vi "Unflatten Asynchronous Execution Units.vi"(8 "error in":errorcluster, 11 "Asynchronous Execution Unit Compiled Information":T4(array[cluster])) -> (0 "error out":errorcluster, 3 "Asynchronous Execution Units":T2(array[cluster]))   [LabVIEW 2020, in "Ballard ARINC 429 Engine.lvlib" / "Custom Device.lvlib"]
uses:
  Custom Device.lvlib
  Asynchronous Execution Unit Compiled Information.ctl
  Asynchronous Execution Unit Runtime Information.ctl
  Interfaces/Execution Unit/Execution Unit.lvclass
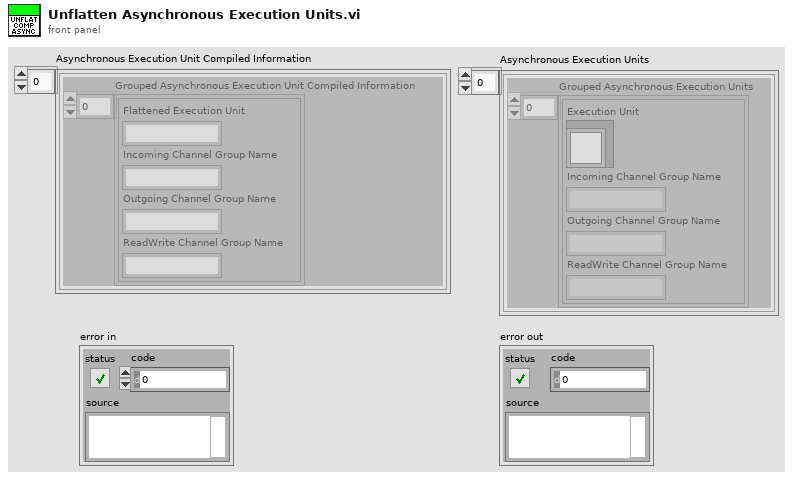
[diagram p1: front panel]
types:
  T1 = typedef "Ballard ARINC 429 Engine.lvlib/Custom Device.lvlib/Asynchronous Execution Unit Runtime Information.ctl" = cluster{"Execution Unit":refnum<class "Execution Unit.lvclass">, "Incoming Channel Group Name":string, "Outgoing Channel Group Name":string, "ReadWrite Channel Group Name":string}
  T2 = cluster{"Grouped Asynchronous Execution Units":T1[]}[]
  T3 = typedef "Ballard ARINC 429 Engine.lvlib/Custom Device.lvlib/Asynchronous Execution Unit Compiled Information.ctl" = cluster{"Flattened Execution Unit":string, "Incoming Channel Group Name":string, "Outgoing Channel Group Name":string, "ReadWrite Channel Group Name":string}
  T4 = cluster{"Grouped Asynchronous Execution Unit Compiled Information":T3[]}[]
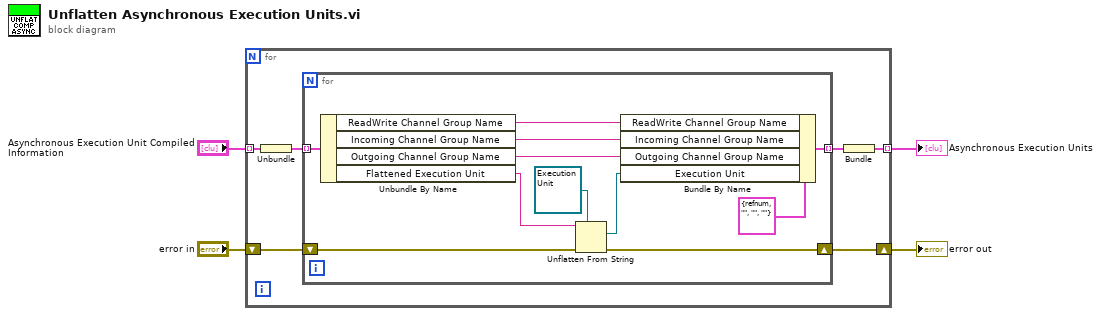
[diagram p0: block diagram]
diagram:
  n1 = for {
    tunnel: "Asynchronous Execution Unit Compiled Information" -> [w8] mode=indexing
    tunnel: [w6] -> w1 mode=indexing
    shift-right: [w9] -> w3
    shift-left: "error in" -> [w10]
    n2 = Unbundle(w8) -> ("Grouped Asynchronous Execution Unit Compiled Information"=w7:T3[])
    n3 = for {
      tunnel: w7 -> [w18] mode=indexing
      tunnel: [w14] -> w5 mode=indexing
      shift-right: [w20] -> w9
      shift-left: w10 -> [w21]
      n4 = Unbundle By Name(w18) -> ("ReadWrite Channel Group Name"=w11:string, "Incoming Channel Group Name"=w13:string, "Outgoing Channel Group Name"=w12:string, "Flattened Execution Unit"=w15:string)
      n5 = Unflatten From String(type=refnum<class "Execution Unit.lvclass"> refnum ("Communication Bus Template Interfaces:Execution Unit.lvlib:Execution Unit.lvclass"), binary string=w15, error in (no error)=w21) -> (value=w16:refnum<class "Execution Unit.lvclass">, error out=w20:errorcluster)  [unwired: 2 in, 1 out]
      n6 = Bundle By Name(cluster=T1 {"Execution Unit"=refnum, "Incoming Channel Group Name"="", "Outgoing Channel Group Name"="", "ReadWrite Channel Group Name"=""} ("Asynchronous Execution Unit Runtime Information"), "ReadWrite Channel Group Name"=w11, "Incoming Channel Group Name"=w13, "Outgoing Channel Group Name"=w12, "Execution Unit"=w16) -> (w14:T1)
    }
    n7 = Bundle(w5) -> (w6:cluster{T1[]})  [unwired: 1 in]
  }
  "error out" <- w3
  "Asynchronous Execution Units" <- w1
